vi "util_launch_criteria.vi"(5 "waitgroup":T2, 7 "change_in_event":refnum<user-event>, 8 "error in (no error)":errorcluster, 9 "recipe_data":variant, 10 "criteria":variant, 11 "criteria_vi_reference":T1) -> (0 "error out":errorcluster)   [LabVIEW 2015, in "lv-recipe-machine.lvlib"]
uses:
  lv-recipe-machine.lvlib
  <userlib>/antonio-alexander/lv-waitgroup/public/_controls/api_waitgroup.ctl
  public/_controls/vi_reference_criteria.ctl
  public/_controls/change.ctl
  <userlib>/antonio-alexander/lv-waitgroup/lv-waitgroup.lvlib
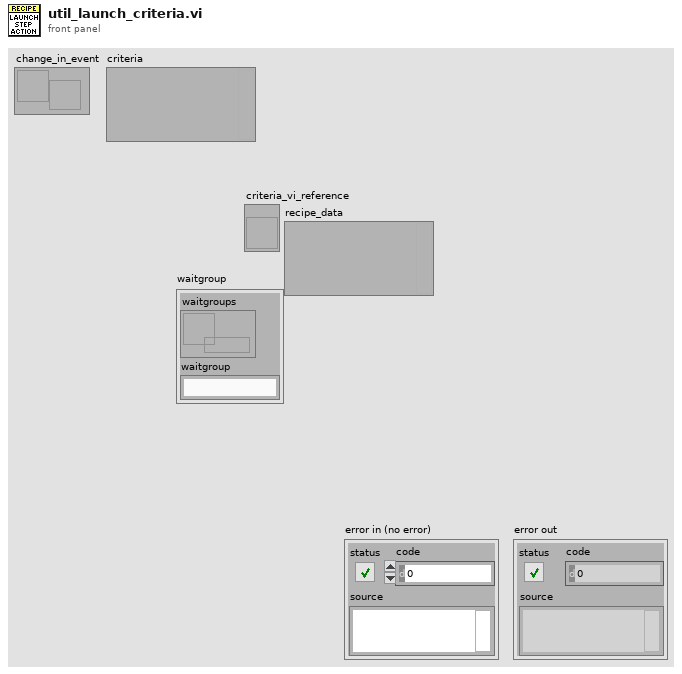
[diagram p1: front panel]
types:
  T1 = typedef "lv-recipe-machine.lvlib/vi_reference_criteria.ctl" = refnum<vi>
  T2 = typedef "lv-waitgroup.lvlib/api_waitgroup.ctl" = cluster{"waitgroups":refnum<data-value>, "waitgroup":string}
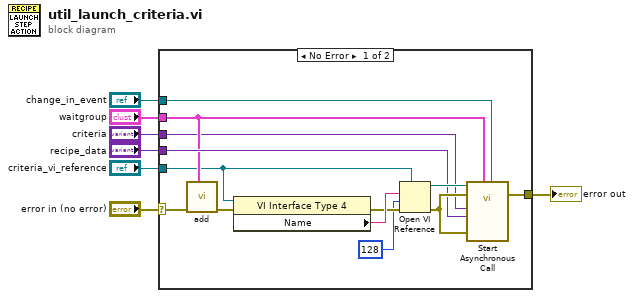
[diagram p0: block diagram]
diagram:
  n1 = case shown="No Error" "error in (no error)" {
    selector: "error in (no error)" -> [w14 w21]
    tunnel: "waitgroup" -> [w11 _]
    tunnel: [w13 w21] -> w5
    tunnel: "criteria_vi_reference" -> [w9 _]
    tunnel: "recipe_data" -> [w12 _]
    tunnel: "change_in_event" -> [w10 _]
    tunnel: "criteria" -> [w8 _]
    frame No Error {
      n2 = call <userlib>:"add.vi"("waitgroup"=w11, "error in (no error)"=w14) -> ("error out"=w19:errorcluster)  [unwired: 9 in]
      n3 = property class="VI Interface Type 4"(reference=w9, error in=w19) -> (error out=w17:errorcluster, "Name"=w18:string)  [unwired: 1 out]
      n4 = Open VI Reference(type specifier VI Refnum (for type only)=w9, vi path=w18, options=128, error in (no error)=w17) -> (vi reference=w16:T1, error out=w20:errorcluster)  [unwired: 2 in]
      n5 = call-by-ref "Start Asynchronous Call"(reference=w16, error in=w20, "change_in_event"=w10, "waitgroup"=w11, 8:"error in (no error)"=w20, "data"=w12, "recipe_data"=w8) -> (error out=w13:errorcluster)  [unwired: 6 in, 2 out]
    }
    frame Error {
    }
  }
  "error out" <- w5
